vi "Persistant Ramp Time DAO.vi"(0 "Ramp Time Actions":T4, 3 "Config Ref Number":T3, 7 "Ramp Time In":T1, 11 "error in (no error)":errorcluster) -> (8 "Ramp Time Out":T1, 14 "Config Ref Number out":T3, 15 "error out":errorcluster)   [LabVIEW 2013]
uses:
  Metadata/Persistant DAO Actions.ctl
  MixedMode/Ramp Time Input.ctl
  MixedMode/Ramp Control.ctl
  <vilib>/Utility/config.llb/Config Data RefNum.ctl
  <vilib>/Utility/config.llb/NI_LVConfig.lvlib
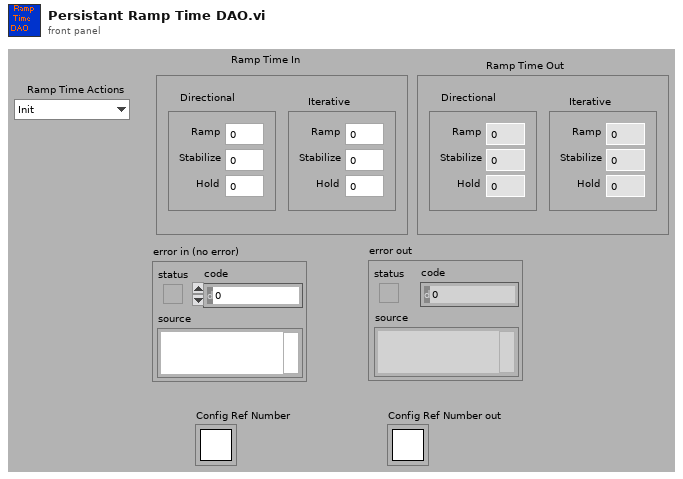
[diagram p1: front panel]
types:
  T1 = typedef "Ramp Time Input.ctl" = cluster{"Directional":T2, "Iterative":T2}
  T2 = typedef "Ramp Control.ctl" = cluster{"Ramp":dbl, "Stabilize":dbl, "Hold":dbl}
  T3 = typedef "NI_LVConfig.lvlib/Config Data RefNum.ctl" = refnum<k1>
  T4 = typedef "Persistant DAO Actions.ctl" = enum16{"Init", "Get", "Set", "Load", "Save"}
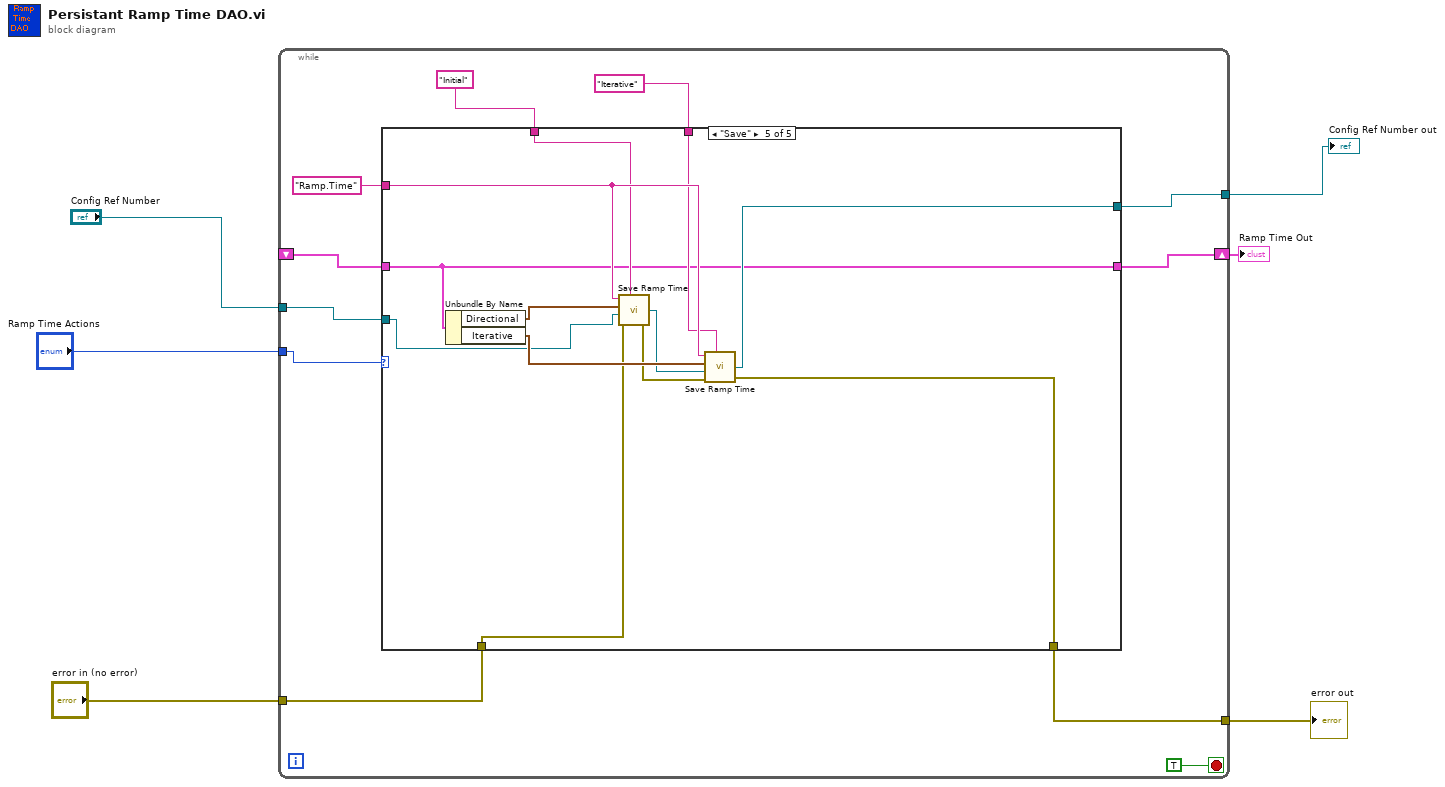
[diagram p0: block diagram]
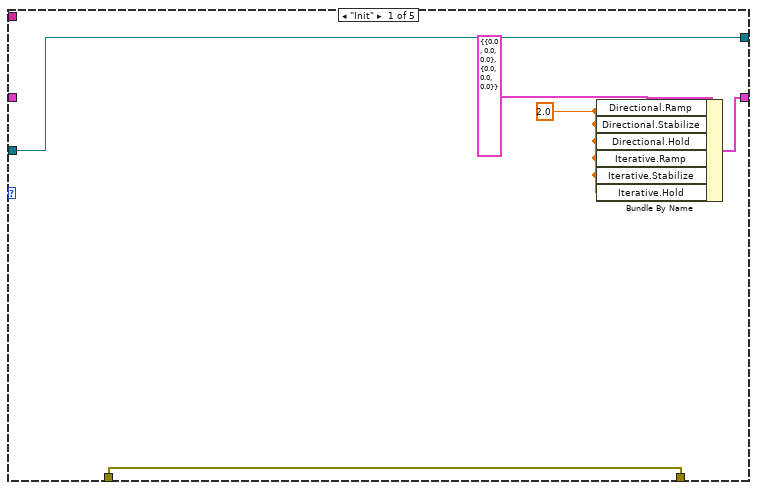
[diagram p2: hidden frame]
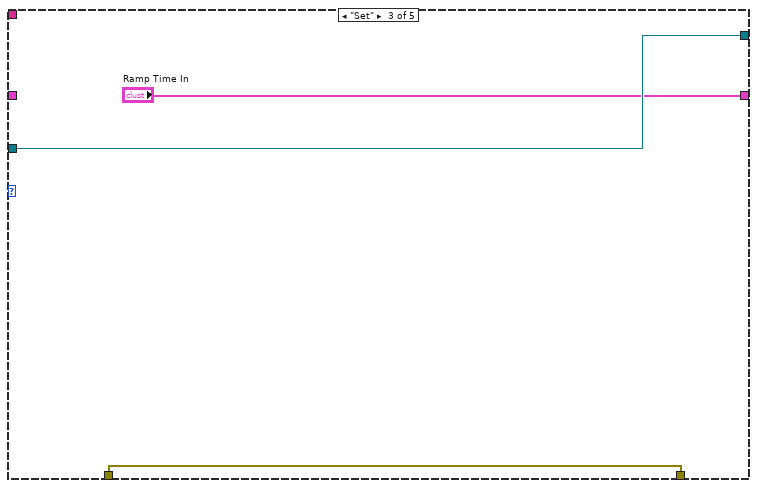
[diagram p4: hidden frame]
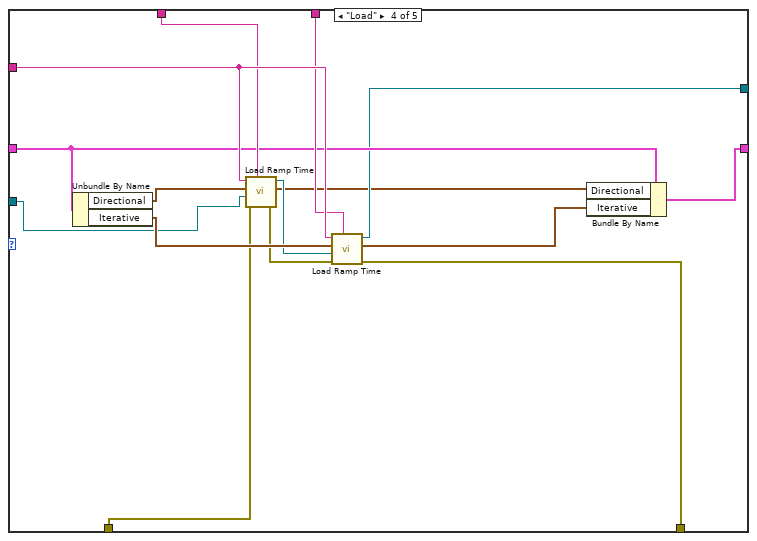
[diagram p5: hidden frame]
diagram:
  n1 = while {
    tunnel: "Ramp Time Actions" -> [w16]
    tunnel: "Config Ref Number" -> [w15]
    tunnel: "error in (no error)" -> [w13]
    tunnel: [w12] -> w3
    shift-right: [w11] -> w1
    shift-left: _ -> [w10]
    tunnel: [w8] -> w2
    stop <- TRUE stop-if-true
    n2 = case shown="\"Save\"" w16 {
      tunnel: "Initial" ("section") -> [_ _ _ w41 w54]
      tunnel: w15 -> [w22 w25 w28 w35 w49]
      tunnel: w13 -> [w21 w23 w26 w31 w47]
      tunnel: [w22 w25 w28 w34 w48] -> w12
      tunnel: [w19 w24 "Ramp Time In" w43 w44] -> w11
      tunnel: w10 -> [_ w24 _ w39 w44]
      tunnel: "Iterative" ("section") -> [_ _ _ w40 w53]
      tunnel: [w21 w23 w26 w29 w45] -> w8
      tunnel: "Ramp.Time" ("section") -> [_ _ _ w42 w55]
      frame "Init" {
        w18 = 2.0 ("Directional.Ramp")
        n3 = Bundle By Name(cluster=T1 {"Directional"={"Ramp"=0.0, "Stabilize"=0.0, "Hold"=0.0}, "Iterative"={"Ramp"=0.0, "Stabilize"=0.0, "Hold"=0.0}} ("Ramp Time In"), "Directional.Ramp"=w18, "Directional.Stabilize"=w18, "Directional.Hold"=w18, "Iterative.Ramp"=w18, "Iterative.Stabilize"=w18, "Iterative.Hold"=w18) -> (w19:T1)
      }
      frame "Get" {
      }
      frame "Set" {
      }
      frame "Load" {
        n4 = Unbundle By Name(w39) -> ("Directional"=w38:T2, "Iterative"=w37:T2)
        n5 = call "Load Ramp Time.vi"("Ramp Type String"=w41, "error in (no error)"=w31, "refnum"=w35, "Input Cluster"=w38, "section"=w42) -> ("error out"=w30:errorcluster, "output cluster"=w32:T2, "refnum out"=w36:T3)  [unwired: 1 out]
        n6 = call "Load Ramp Time.vi"("Ramp Type String"=w40, "error in (no error)"=w30, "refnum"=w36, "Input Cluster"=w37, "section"=w42) -> ("error out"=w29:errorcluster, "output cluster"=w33:T2, "refnum out"=w34:T3)  [unwired: 1 out]
        n7 = Bundle By Name(cluster=w39, "Directional"=w32, "Iterative"=w33) -> (w43:T1)
      }
      frame "Save" {
        n8 = Unbundle By Name(w44) -> ("Directional"=w52:T2, "Iterative"=w51:T2)
        n9 = call "Save Ramp Time.vi"("section"=w55, "Input Cluster"=w52, "refnum"=w49, "error in (no error)"=w47, "Ramp Type String"=w54) -> ("refnum out"=w50:T3, "error out"=w46:errorcluster)  [unwired: 1 out]
        n10 = call "Save Ramp Time.vi"("section"=w55, "Input Cluster"=w51, "refnum"=w50, "error in (no error)"=w46, "Ramp Type String"=w53) -> ("refnum out"=w48:T3, "error out"=w45:errorcluster)  [unwired: 1 out]
      }
    }
  }
  "error out" <- w2
  "Config Ref Number out" <- w3
  "Ramp Time Out" <- w1
